vi "FF_GenAssistveForceVector.vi"(2 "AnkleInGCS":dbl[](array[numeric]), 3 "Cloest Point on Traj":T1) -> (0 "Closest Point in GCS":dbl[](array[numeric]), 1 "Assist Force NTD":T2)   [LabVIEW 2016, in "ForceField.lvclass"]
uses:
  ForceField.lvclass
  TypeDef/ForceNTD.ctl
  TypeDef/AnkleTrajPt.ctl
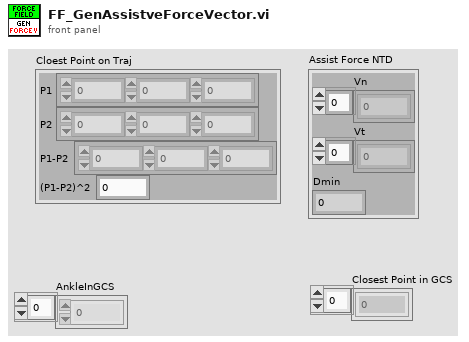
[diagram p1: front panel]
types:
  T1 = typedef "ForceField.lvclass/AnkleTrajPt.ctl" = cluster{"P1":dbl[], "P2":dbl[], "P1-P2":dbl[], "(P1-P2)^2":dbl}
  T2 = typedef "ForceField.lvclass/ForceNTD.ctl" = cluster{"Vn":dbl[], "Vt":dbl[], "Dmin":dbl}
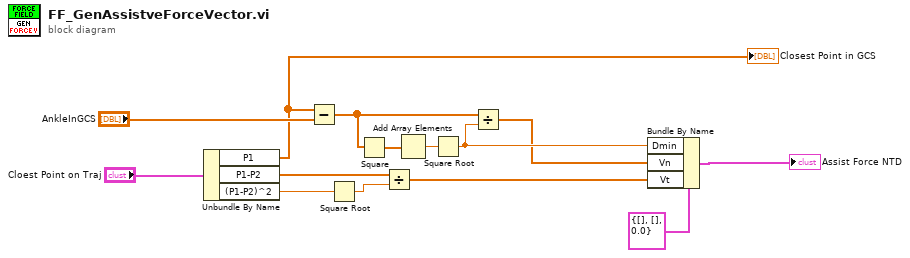
[diagram p0: block diagram]
diagram:
  n1 = Unbundle By Name("Cloest Point on Traj") -> ("P1"=w11:dbl[], "P1-P2"=w13:dbl[], "(P1-P2)^2"=w3:dbl)
  "Closest Point in GCS" <- w11
  n2 = Subtract(x=w11, y="AnkleInGCS") -> (x-y=w6:dbl[])
  n3 = Square Root(x=w3) -> (sqrt(x)=w2:dbl)
  n4 = Square(x=w6) -> (x^2=w4:dbl[])
  n5 = Divide(x=w13, y=w2) -> (x/y=w8:dbl[])
  n6 = Add Array Elements(numeric array=w4) -> (sum=w5:dbl)
  n7 = Square Root(x=w5) -> (sqrt(x)=w14:dbl)
  n8 = Divide(x=w6, y=w14) -> (x/y=w7:dbl[])
  n9 = Bundle By Name(cluster=T2 {"Vn"=[], "Vt"=[], "Dmin"=0.0} ("TND"), "Dmin"=w14, "Vn"=w7, "Vt"=w8) -> (→"Assist Force NTD":T2)
